vi "IT-M7700 DC Voltage Output.vi"() -> ()   [LabVIEW 2015]
doc: "This example shows how to configure the instrument's output voltage level, over current protection, and over voltage protection. The actual voltage level and actual current level are returned as well as whether over voltage protection (OVP) or over current protection (OCP) has been tripped."
uses:
  <instrlib>/IT-M7700/IT-M7700.lvlib
panel:
  in  "OCP RMS Level(A)":dbl min=0.0 format="%.2g"
  in  "DC Voltage(V)":dbl min=0.0 format="%.2g"
  in  "?":bool
  out "Read Power(W)":dbl format="%.3g"
  out "Read DC Current(A)":dbl format="%.3g"
  out "Read DC Voltage(V)":dbl format="%.3g"
  in  "Serial Configuration":T1={"Baud Rate"=9600, "Parity"=0, "Data Bits"=8, "Stop Bits"=10, "Flow Control"=0} {"Flow Control" items=["None", "XON/XOFF", "RTS/CTS", "XON/XOFF & RTS/CTS", "DTR/DSR", "XON/XOFF & DTR/DSR"]; "Stop Bits" items=["1.0"=10, "1.5"=15, "2.0"=20]; "Data Bits" items=["7"=7, "8"=8]; "Parity" items=["None", "Odd", "Even", "Mark", "Space"]; "Baud Rate" items=["1200"=1200, "2400"=2400, "4800"=4800, "9600"=9600, "19200"=19200, "34800"=34800, "57600"=57600, "115200"=115200]}
  in  "VISA resource name":refnum<visa-resource-name>
  # "Source DC Output"
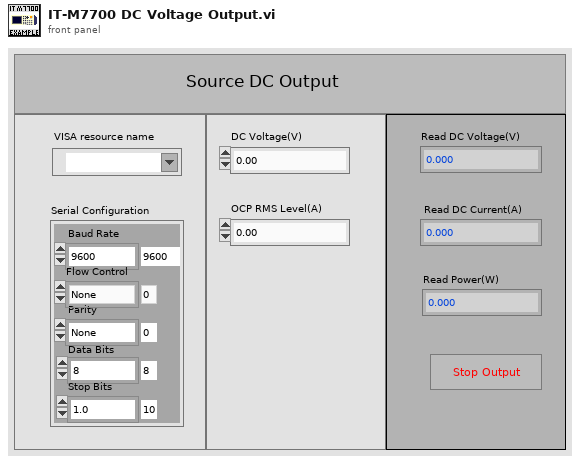
[diagram p1: front panel]
types:
  T1 = cluster{"Baud Rate":u32, "Parity":u16, "Data Bits":u16, "Stop Bits":u16, "Flow Control":u16}
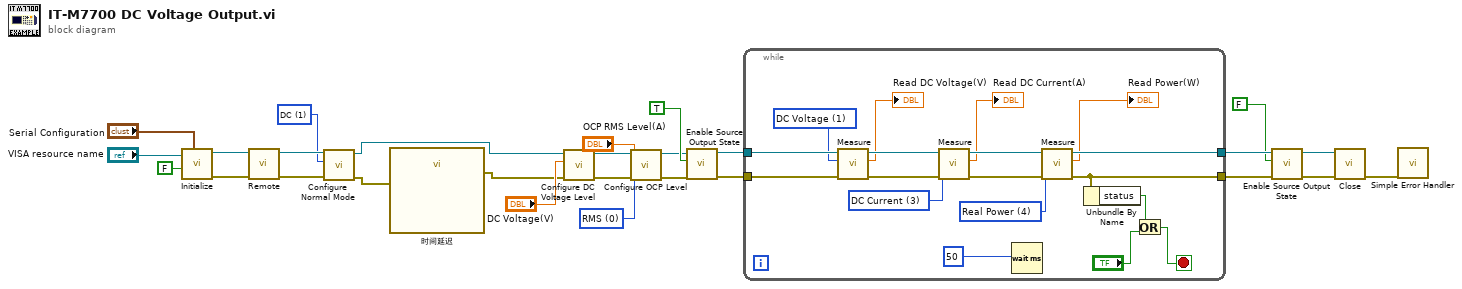
[diagram p0: block diagram]
diagram:
  w2 = u16 0 items=["RMS", "PEAK"] ("Type")
  w21 = u16 1 items=["AC", "DC", "AC+DC"] ("Mode")
  n1 = call <instrlib>:"Initialize.vi"("Serial Configuration"="Serial Configuration", "Reset"=FALSE, "VISA resource name"="VISA resource name") -> ("error out"=w25:errorcluster, "VISA resource name out"=w26:refnum<visa-resource-name>)  [unwired: 7 in]
  n2 = call <instrlib>:"Remote.vi"("error in"=w25, "VISA resource name"=w26) -> ("error out"=w22:errorcluster, "VISA resource name out"=w23:refnum<visa-resource-name>)  [unwired: 8 in]
  n3 = call <instrlib>:"Configure Normal Mode.vi"("error in"=w22, "Mode"=w21, "VISA resource name"=w23) -> ("error out"=w9:errorcluster, "VISA resource name out"=w10:refnum<visa-resource-name>)  [unwired: 7 in]
  n4 = call "时间延迟"("error in (no error)"=w9) -> ("error out"=w8:errorcluster)  [unwired: 10 in]
  n5 = call <instrlib>:"Configure DC Voltage Level.vi"("error in"=w8, "Level(V)"="DC Voltage(V)", "VISA resource name"=w10) -> ("error out"=w5:errorcluster, "VISA resource name out"=w6:refnum<visa-resource-name>)  [unwired: 7 in]
  n6 = call <instrlib>:"Configure OCP Level.vi"("error in"=w5, "Level(A)"="OCP RMS Level(A)", "Type"=w2, "VISA resource name"=w6) -> ("error out"=w4:errorcluster, "VISA resource name out"=w3:refnum<visa-resource-name>)  [unwired: 6 in]
  n7 = call <instrlib>:"Enable Source Output State.vi"("error in"=w4, "State"=TRUE, "VISA resource name"=w3) -> ("error out"=w19:errorcluster, "VISA resource name out"=w18:refnum<visa-resource-name>)  [unwired: 7 in]
  n8 = while {
    tunnel: w18 -> [w45]
    tunnel: w19 -> [w44]
    tunnel: [w39] -> w16
    tunnel: [w29] -> w15
    stop <- w30 stop-if-true
    w32 = u16 4 items=["AC Voltage", "DC Voltage", "AC Current", "DC Current", "Real Power", "Apparent Power", "Pfactor Power", "Frequency", "THD", "Current THD", "Reactive Power"] ("Measure Type")
    w33 = u16 3 items=["AC Voltage", "DC Voltage", "AC Current", "DC Current", "Real Power", "Apparent Power", "Pfactor Power", "Frequency", "THD", "Current THD", "Reactive Power"] ("Measure Type")
    w34 = u16 1 items=["AC Voltage", "DC Voltage", "AC Current", "DC Current", "Real Power", "Apparent Power", "Pfactor Power", "Frequency", "THD", "Current THD", "Reactive Power"] ("Measure Type")
    n9 = call <instrlib>:"Measure.vi"("error in"=w44, "Measure Type"=w34, "VISA resource name"=w45) -> ("error out"=w42:errorcluster, "Measurement"=→"Read DC Voltage(V)":dbl, "VISA resource name out"=w43:refnum<visa-resource-name>)  [unwired: 6 in]
    n10 = call <instrlib>:"Measure.vi"("error in"=w42, "Measure Type"=w33, "VISA resource name"=w43) -> ("error out"=w40:errorcluster, "Measurement"=→"Read DC Current(A)":dbl, "VISA resource name out"=w41:refnum<visa-resource-name>)  [unwired: 6 in]
    n11 = Wait (ms)(milliseconds to wait=50) -> ()  [unwired: 1 out]
    n12 = call <instrlib>:"Measure.vi"("error in"=w40, "Measure Type"=w32, "VISA resource name"=w41) -> ("error out"=w29:errorcluster, "Measurement"=→"Read Power(W)":dbl, "VISA resource name out"=w39:refnum<visa-resource-name>)  [unwired: 6 in]
    n13 = Unbundle By Name(w29) -> ("status"=w28:bool)
    n14 = Or(x=w28, y="?") -> (x .or. y?=w30:bool)
  }
  n15 = call <instrlib>:"Enable Source Output State.vi"("error in"=w15, "State"=FALSE, "VISA resource name"=w16) -> ("error out"=w14:errorcluster, "VISA resource name out"=w13:refnum<visa-resource-name>)  [unwired: 7 in]
  n16 = call <instrlib>:"Close.vi"("error in"=w14, "VISA resource name"=w13) -> ("error out"=w24:errorcluster)  [unwired: 9 in]
  n17 = call <vilib>:"Simple Error Handler.vi"("error in (no error)"=w24) -> ()  [unwired: 4 in, 5 out]
